vi "testExample 4.vi"(8 "error in (no error)":errorcluster, 11 "TestCase in":refnum<class "ReadADC.lvclass">) -> (0 "error out":errorcluster, 3 "TestCase out":refnum<class "ReadADC.lvclass">)   [LabVIEW 2020, in "ReadADC.lvclass"]
uses:
  ReadADC.lvclass
  <vilib>/addons/_JKI Toolkits/VI Tester/TestCase.llb/TestCase.lvclass
  C:/Program Files (x86)/National Instruments/LabVIEW 2020/vi.lib/addons/_JKI Toolkits/VI Tester/TestCase.llb/TestCase.lvclass
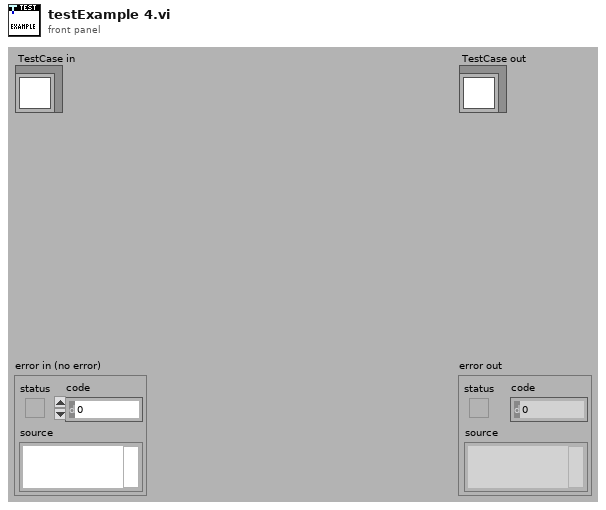
[diagram p1: front panel]
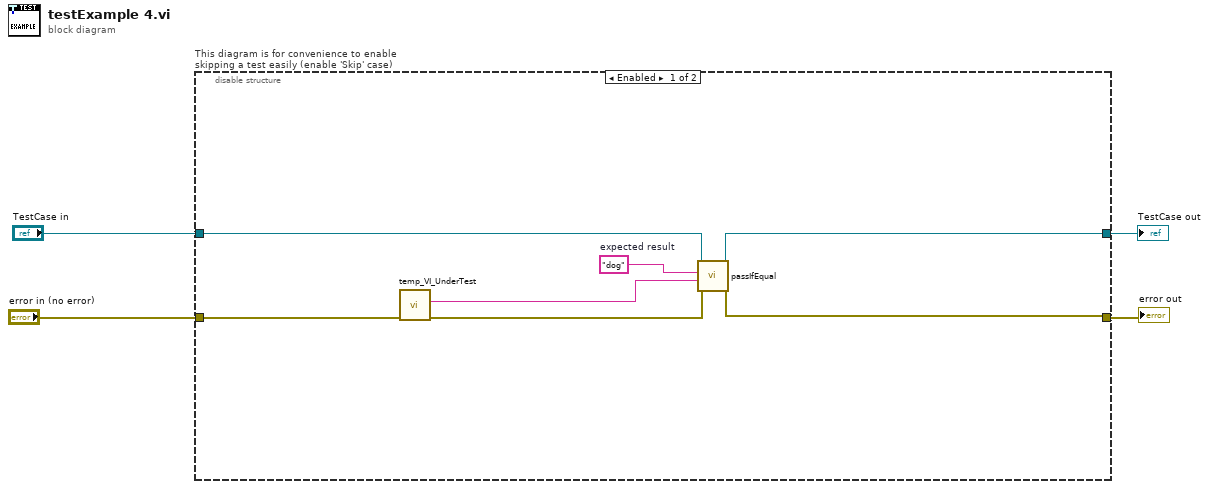
[diagram p0: block diagram]
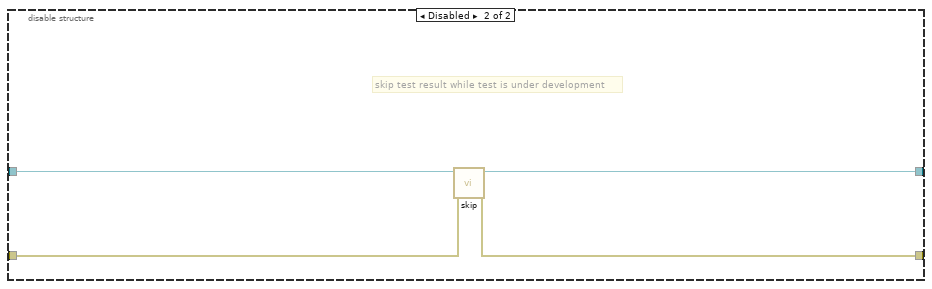
[diagram p2: hidden frame]
diagram:
  n1 = disable-structure "This diagram is for convenience to enable skipping a test easily (enable 'Skip' case)" shown="Enabled" {
    disable-tunnel: "TestCase in" -> [w10 w15]
    disable-tunnel: [w9 w13] -> w1
    disable-tunnel: [w8 w14] -> w3
    disable-tunnel: "error in (no error)" -> [w7 w12]
    frame Enabled {
      w11 = "dog"  # expected result
      n2 = call "temp_VI_UnderTest.vi"("error in"=w7) -> ("error out"=w6:errorcluster, "actual result"=w5:string)  [unwired: 9 in]
      n3 = call-dynamic "passIfEqual.vi"("error in (no error)"=w6, "y"=w5, "x"=w11, "TestCase in"=w10) -> ("error out"=w8:errorcluster, "TestCase out"=w9:refnum<class "ReadADC.lvclass">)  [unwired: 6 in]
    }
    frame Disabled {
      # "skip test result while test is under development"
      n4 = call <vilib>:"skip.vi"("error in (no error)"=w12, "TestCase in"=w15) -> ("error out"=w14:errorcluster, "TestCase out"=w13:refnum<class "ReadADC.lvclass">)  [unwired: 8 in]
    }
  }
  "error out" <- w3
  "TestCase out" <- w1
